vi "AH 2550 Self Test.vi"() -> ()   [LabVIEW 2016]
doc: "This example shows how to configure the bridge to run a self-test and create a report file containing the results."
uses:
  Andeen-Hagerling 2550.lvlib
panel:
  in  "Log Results\nto File":bool
  out "Self-Test Results":string
  in  "VISA resource name":refnum<visa-resource-name>
  in  "Serial Configuration":T1={"Baud Rate"=9600, "Parity"=0, "Data Bits"=8, "Stop Bits"=10} {"Stop Bits" items=["1.0"=10, "1.5"=15, "2.0"=20]; "Data Bits" items=["7"=7, "8"=8]; "Parity" items=["None", "Odd", "Even", "Mark", "Space"]; "Baud Rate" items=["300"=300, "600"=600, "1200"=1200, "2400"=2400, "4800"=4800, "9600"=9600, "19200"=19200]}
  # "AH 2550A ULTRA-PRECISION 1kHz CAPACITANCE BRIDGE"
  # "Self Test"
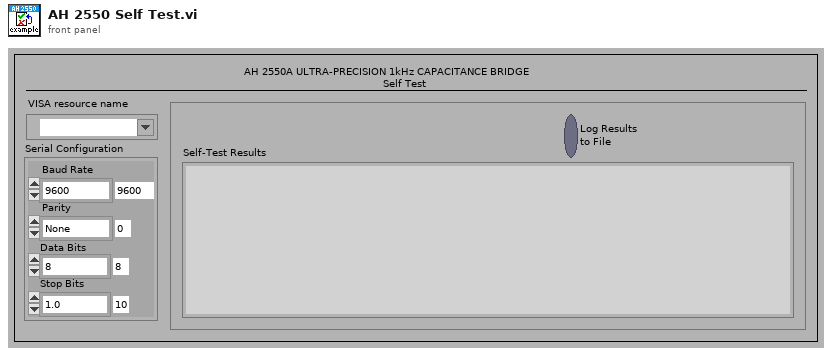
[diagram p1: front panel]
types:
  T1 = cluster{"Baud Rate":u32, "Parity":u16, "Data Bits":u16, "Stop Bits":u16}
  T2 = enum16{"open", "replace", "create", "open or create", "replace or create", "replace or create with confirmation"}
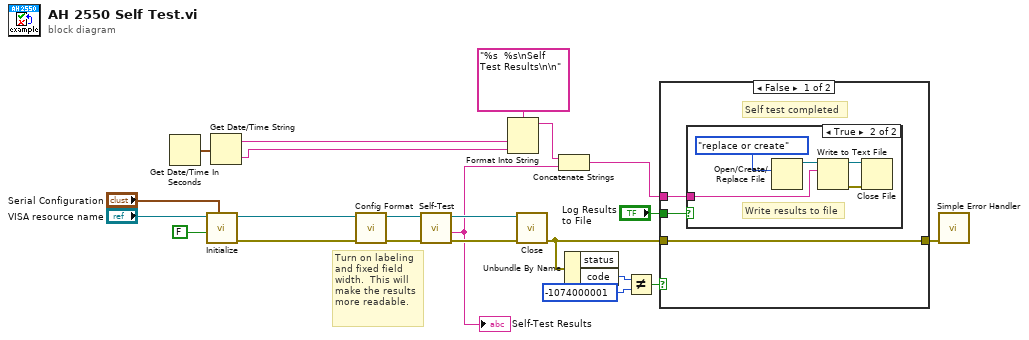
[diagram p0: block diagram]
diagram:
  # "Turn on labeling\nand fixed field\nwidth.  This will\nmake the results\nmore readable."
  n1 = Get Date/Time In Seconds() -> (seconds since 1Jan1904=w6:timestamp)
  n2 = call "Initialize.vi"("Serial Configuration"="Serial Configuration", "Reset (True)"=FALSE, "VISA resource name"="VISA resource name") -> ("error out"=w2:errorcluster, "VISA resource name out"=w3:refnum<visa-resource-name>)  [unwired: 7 in]
  n3 = Get Date/Time String(seconds (now)=w6) -> (date string=w5:string, time string=w4:string)  [unwired: 2 in]
  n4 = call "Config Format.vi"("error in"=w2, "VISA resource name"=w3) -> ("error out"=w17:errorcluster, "VISA resource name out"=w18:refnum<visa-resource-name>)  [unwired: 8 in]
  n5 = call "Self-Test.vi"("error in (no error)"=w17, "VISA resource name"=w18) -> ("error out"=w19:errorcluster, "Self-Test Result"=w9:string, "VISA resource name out"=w20:refnum<visa-resource-name>)  [unwired: 6 in, 1 out]
  "Self-Test Results" <- w9
  n6 = Format Into String(format string="%s  %s\nSelf Test Results\n\n", w5, w4) -> (resulting string=w8:string)  [unwired: 2 in, 1 out]
  n7 = call "Close.vi"("error in (no error)"=w19, "VISA resource name"=w20) -> ("error out"=w11:errorcluster)  [unwired: 9 in]
  n8 = Concatenate Strings(w8, w9) -> (w7:string)
  n9 = Unbundle By Name(w11) -> ("code"=w16:i32)  [unwired: 1 out]
  n10 = Not Equal?(x=w16, y=-1074000001 ("Code")) -> (x != y?=w14:bool)
  n11 = case shown="False" w14 {
    tunnel: "Log Results\nto File" -> [w23 _]
    tunnel: [w25 w31] -> w12
    tunnel: w11 -> [w25 w31]
    tunnel: w7 -> [w24 _]
    frame False {
      # "Self test completed"
      n12 = case shown="True" w23 {
        tunnel: w24 -> [_ w28]
        frame False {
        }
        frame True {
          # "Write results to file"
          n13 = Open/Create/Replace File(operation (0:open)=T2."replace or create") -> (refnum out=w29:refnum<file>)  [unwired: 5 in, 2 out]
          n14 = Write to Text File(file (use dialog)=w29, text=w28) -> (refnum out=w26:refnum<file>, error out=w27:errorcluster)  [unwired: 2 in, 1 out]
          n15 = Close File(refnum=w26, error in=w27) -> ()  [unwired: 2 out]
        }
      }
    }
    frame True {
      # "Self test did not complete.  It encountered an\nerror other than \"self-test failed\"."
    }
  }
  n16 = call <vilib>:"Simple Error Handler.vi"("error in (no error)"=w12) -> ()  [unwired: 4 in, 5 out]
